vi "队列堆栈（Key Info）.vi"(8 "error in (no error)":errorcluster caption="错误输入（无错误）", 9 "堆栈操作":T3, 10 "堆栈长度":i32=-1, 11 "入栈元素":T2(ring)=enum."RIGHT" caption="按键类型3") -> (0 "error out":errorcluster caption="错误输出", 1 "堆栈空":bool, 2 "入栈所有元素":T1(array[ring]), 3 "出栈元素":T2(ring)=enum."RIGHT" caption="按键类型3")   [LabVIEW 2012]
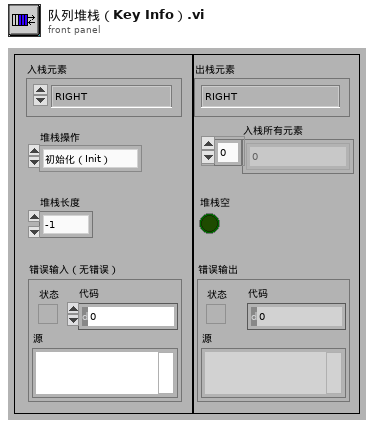
[diagram p1: front panel]
types:
  T1 = enum16{"0", "1", "2", "3", "4", "5", "6", "7", "8", "9", "A", "B", "C", "D", "E", "F", "G", "H", "I", "J", "K", "L", "M", "N", "O", "P", "Q", "R", "S", "T", "U", "V", "W", "X", "Y", "Z", "F1", "F2", "F3", "F4", "F5", "F6", "F7", "F8", "F9", "F10", "F11", "F12", "F13", "F14", "F15", "ADD", "BACK", "BACKSLASH", "CAPITAL", "COMMA", "DECIMAL", "DELETE", "DIVIDE", "DOWN", "END", "EQUALS", "ESCAPE", "GRAVE (`)", "HOME", "INSERT", "LBRACKET", "LCONTROL", "LEFT", "L ALT", "LSHIFT", "LWIN", "MINUS", "MULTIPLY", "NEXT", "NUMLOCK", "NUMPAD_0", "NUMPAD_1", "NUMPAD_2", "NUMPAD_3", "NUMPAD_4", "NUMPAD_5", "NUMPAD_6", "NUMPAD_7", "NUMPAD_8", "NUMPAD_9", "PAUSE", "PERIOD", "PRIOR (PG UP)", "RBRACKET", "RCONTROL", "RETURN", "RIGHT", "R ALT", "RSHIFT", "RWIN", "SCROLL", "SEMICOLON", "SLASH", "SPACE", "SUBTRACT", "TAB", "UP", "ENTER (num pad)", "' (quote)"}[]
  T2 = enum16{"0", "1", "2", "3", "4", "5", "6", "7", "8", "9", "A", "B", "C", "D", "E", "F", "G", "H", "I", "J", "K", "L", "M", "N", "O", "P", "Q", "R", "S", "T", "U", "V", "W", "X", "Y", "Z", "F1", "F2", "F3", "F4", "F5", "F6", "F7", "F8", "F9", "F10", "F11", "F12", "F13", "F14", "F15", "ADD", "BACK", "BACKSLASH", "CAPITAL", "COMMA", "DECIMAL", "DELETE", "DIVIDE", "DOWN", "END", "EQUALS", "ESCAPE", "GRAVE (`)", "HOME", "INSERT", "LBRACKET", "LCONTROL", "LEFT", "L ALT", "LSHIFT", "LWIN", "MINUS", "MULTIPLY", "NEXT", "NUMLOCK", "NUMPAD_0", "NUMPAD_1", "NUMPAD_2", "NUMPAD_3", "NUMPAD_4", "NUMPAD_5", "NUMPAD_6", "NUMPAD_7", "NUMPAD_8", "NUMPAD_9", "PAUSE", "PERIOD", "PRIOR (PG UP)", "RBRACKET", "RCONTROL", "RETURN", "RIGHT", "R ALT", "RSHIFT", "RWIN", "SCROLL", "SEMICOLON", "SLASH", "SPACE", "SUBTRACT", "TAB", "UP", "ENTER (num pad)", "' (quote)"}
  T3 = typedef "堆栈操作.ctl" = enum16{"初始化（Init）", "进栈（Push）", "出栈（Pop）", "状态（Status)", "释放"}
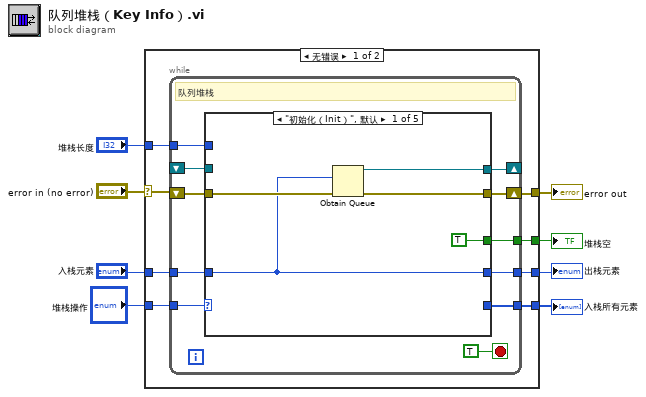
[diagram p0: block diagram]
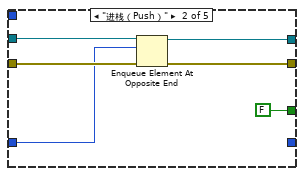
[diagram p2: hidden frame]
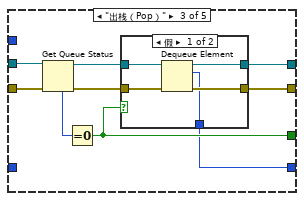
[diagram p3: hidden frame]
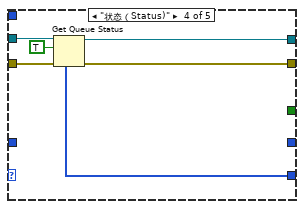
[diagram p5: hidden frame]
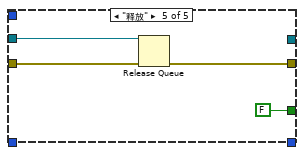
[diagram p6: hidden frame]
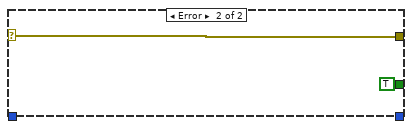
[diagram p7: hidden frame]
diagram:
  n1 = case shown="无错误" "error in (no error)" {
    selector: "error in (no error)" -> [w12 w66]
    tunnel: [w11 w66] -> w7
    tunnel: "堆栈操作" -> [w16 _]
    tunnel: "入栈元素" -> [w15 _]
    tunnel: [w14 _] -> w2
    tunnel: "堆栈长度" -> [w13 _]
    tunnel: [w10 TRUE] -> w4
    tunnel: [w9 _] -> w1
    frame No Error {
      n2 = while {
        tunnel: w16 -> [w27]
        tunnel: w15 -> [w26]
        tunnel: [w25] -> w14
        tunnel: w13 -> [w24]
        shift-right: [w21] -> w11
        shift-left: w12 -> [w22]
        shift-right: [w20] -> _
        shift-left: _ -> [w19]
        tunnel: [w18] -> w10
        tunnel: [w17] -> w9
        stop <- TRUE stop-if-true
        # "队列堆栈"
        n3 = case shown="\"初始化（Init）\", 默认" w27 {
          tunnel: w26 -> [w29 w34 _ _ _]
          tunnel: [w29 _ w39 _ _] -> w25
          tunnel: w24 -> [_ _ _ _ _]
          tunnel: w22 -> [w32 w38 w47 w59 w64]
          tunnel: [w31 w37 w40 w56 w63] -> w21
          tunnel: [w30 w35 w42 w57 _] -> w20
          tunnel: w19 -> [_ w36 w46 w60 w62]
          tunnel: [TRUE FALSE w44 _ FALSE] -> w18
          tunnel: [_ _ _ w55 _] -> w17
          frame "初始化（Init）", Default {
            n4 = Obtain Queue(element data type=w29, error in (no error)=w32) -> (queue out=w30:refnum<queue>, error out=w31:errorcluster)  [unwired: 3 in, 1 out]
          }
          frame "进栈（Push）" {
            n5 = Enqueue Element At Opposite End(queue=w36, element=w34, error in (no error)=w38) -> (queue out=w35:refnum<queue>, error out=w37:errorcluster)  [unwired: 1 in, 1 out]
          }
          frame "出栈（Pop）" {
            n6 = Get Queue Status(queue=w46, error in (no error)=w47) -> (queue out=w43:refnum<queue>, error out=w41:errorcluster, # elements in queue=w45:i32)  [unwired: 1 in, 5 out]
            n7 = Equal To 0?(x=w45) -> (x = 0?=w44:bool)
            n8 = case shown="假" w44 {
              tunnel: w43 -> [w52 w54]
              tunnel: [w51 w54] -> w42
              tunnel: w41 -> [w50 w53]
              tunnel: [w49 w53] -> w40
              tunnel: [w48 _] -> w39
              frame False {
                n9 = Dequeue Element(queue=w52, error in (no error)=w50) -> (queue out=w51:refnum<queue>, element=w48:T2, error out=w49:errorcluster)  [unwired: 1 in, 1 out]
              }
              frame True {
              }
            }
          }
          frame "状态（Status)" {
            n10 = Get Queue Status(queue=w60, return elements? (F)=TRUE ("返回元素？(F)"), error in (no error)=w59) -> (queue out=w57:refnum<queue>, error out=w56:errorcluster, elements=w55:T1)  [unwired: 5 out]
          }
          frame "释放" {
            n11 = Release Queue(queue=w62, error in (no error)=w64) -> (error out=w63:errorcluster)  [unwired: 1 in, 2 out]
          }
        }
      }
    }
    frame Error {
    }
  }
  "error out" <- w7
  "堆栈空" <- w4
  "出栈元素" <- w2
  "入栈所有元素" <- w1
